vi "Clear Data.vi"(0 "VISA resource name":refnum<visa-resource-name>, 5 "Clear Security Setting (False)":bool, 7 "Clear Setting Except Security (False)":bool, 9 "Clear Data, Summary, Log (False)":bool, 11 "error in (no error)":errorcluster) -> (4 "VISA resource name out":refnum<visa-resource-name>, 15 "error out":errorcluster)   [LabVIEW 2020, in "Yokogawa GX Series.lvlib"]
doc: "Clears the measured, computed data, and initializes setup data."
uses:
  <instrlib>/Yokogawa GX Series/Yokogawa GX Series.lvlib
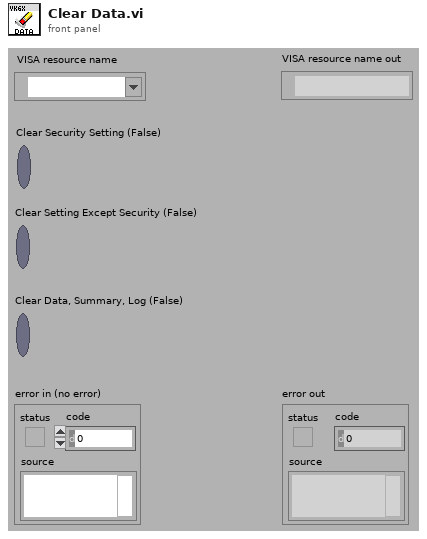
[diagram p1: front panel]
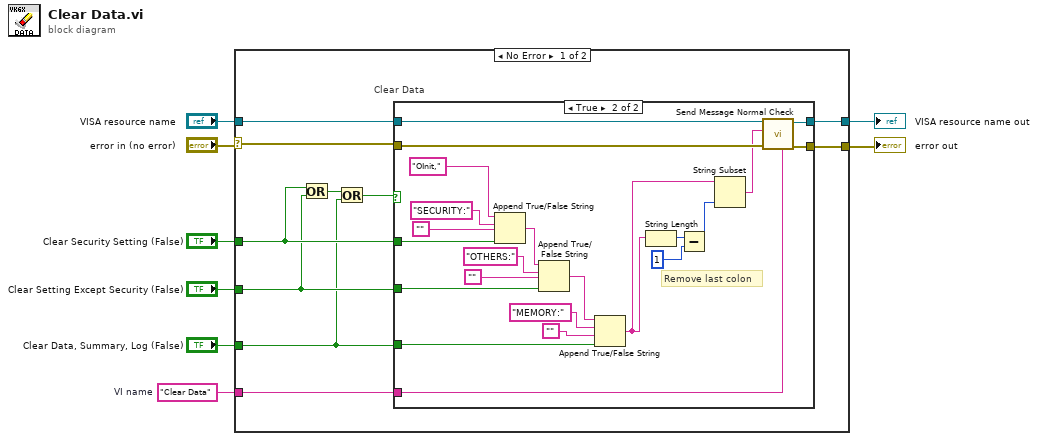
[diagram p0: block diagram]
diagram:
  w2 = "Clear Data"  # VI name
  n1 = case shown="No Error" "error in (no error)" {
    selector: "error in (no error)" -> [w9 w43]
    tunnel: "Clear Security Setting (False)" -> [w16 _]
    tunnel: "Clear Setting Except Security (False)" -> [w15 _]
    tunnel: "Clear Data, Summary, Log (False)" -> [w14 _]
    tunnel: [w13 w44] -> w5
    tunnel: [w12 w43] -> w4
    tunnel: "VISA resource name" -> [w11 w44]
    tunnel: w2 -> [w10 _]
    frame No Error {
      # "Clear Data"
      n2 = Or(x=w16, y=w15) -> (x .or. y?=w18:bool)
      n3 = Or(x=w18, y=w14) -> (x .or. y?=w17:bool)
      n4 = case shown="True" w17 {
        tunnel: w16 -> [_ w32]
        tunnel: w15 -> [_ w29]
        tunnel: w14 -> [_ w26]
        tunnel: [w20 w42] -> w13
        tunnel: [w19 w35] -> w12
        tunnel: w11 -> [w20 w41]
        tunnel: w9 -> [w19 w40]
        tunnel: w10 -> [_ w25]
        frame False {
        }
        frame True {
          # "Remove last colon"
          n5 = Append True/False String(1:w32, 2:"", 3:"SECURITY:", 4:"OInit,") -> (0:w31:string)
          n6 = Append True/False String(1:w29, 2:"", 3:"OTHERS:", 4:w31) -> (0:w28:string)
          n7 = Append True/False String(1:w26, 2:"", 3:"MEMORY:", 4:w28) -> (0:w22:string)
          n8 = String Length(string=w22) -> (length=w38:i32)
          n9 = Subtract(x=w38, y=1) -> (x-y=w36:i32)
          n10 = String Subset(string=w22, length (rest)=w36) -> (substring=w39:string)  [unwired: 1 in]
          n11 = call <instrlib>:"Send Message Normal Check.vi"("Source (\"\")"=w25, "error in (no error)"=w40, "Send Message (\"\")"=w39, "VISA resource name"=w41) -> ("error out"=w35:errorcluster, "VISA resource name out"=w42:refnum<visa-resource-name>)  [unwired: 2 in, 4 out]
        }
      }
    }
    frame Error {
    }
  }
  "error out" <- w4
  "VISA resource name out" <- w5
